vi "exec.vi"(8 "error in (no error)":errorcluster, 10 "context":refnum<class "Context.lvclass">, 11 "Start in":refnum<class "Start.lvclass">) -> (0 "error out":errorcluster, 2 "context 2":refnum<class "Context.lvclass">, 3 "Start out":refnum<class "Start.lvclass">)   [LabVIEW 2013, in "Start.lvclass"]
uses:
  Start.lvclass
  Context/Context.lvclass
  Start.lvclass/Start.ctl
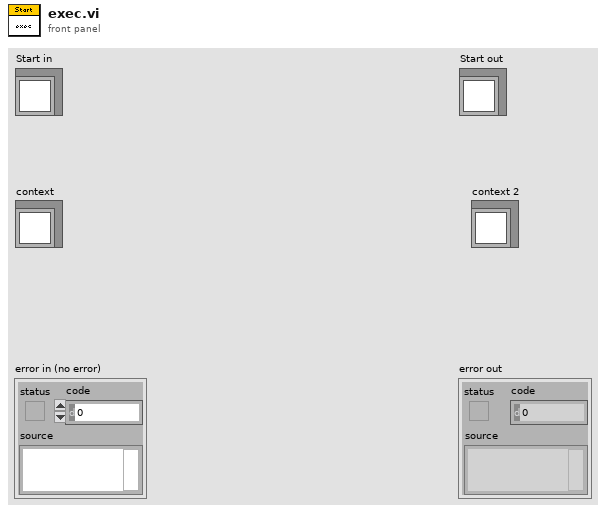
[diagram p1: front panel]
types:
  T1 = typedef "ILCAppConfig.ctl" = cluster{"ILCConfig":T2, "SerialConfig":T5, "Application Timing":T7}
  T2 = typedef "ILCCommon.lvlib/ILCConfiguration.lvlib/ILCConfig.ctl" = cluster{"Input Channels":T3, "Scan Rate (Hz) ":T4, "ADC PGA Gain":u8}
  T3 = typedef "ILCCommon.lvlib/ILCConfiguration.lvlib/InputChannels.ctl" = enum16{"Channel 0", "3 Channels", "5 Channels"}
  T4 = typedef "ILCCommon.lvlib/ILCConfiguration.lvlib/ScanRate_Hz_MultichannelOptions.ctl" = enum16{"50", "60", "100", "120", "200", "240", "300", "400", "480", "600", "1200", "2400", "4800"}
  T5 = typedef "SerialProtocols.lvlib/SerialConfig.ctl" = cluster{"VISA resource name":refnum<visa-resource-name>, "Baud Rate":u32, "Data Bits":u16, "Parity":enum16{"None", "Odd", "Even", "Mark", "Space"}, "Stop Bits":u16, "Flow Control":u16, "Timeout (ms)":u32, "Serial Protocol":T6}
  T6 = typedef "SerialProtocols.lvlib/SerialProtocol.ctl" = enum16{"RS232", "RS485", "SerialSimulator"}
  T7 = typedef "Application.lvlib/ApplicationTiming.ctl" = cluster{"Loop Period (ms)":u16}
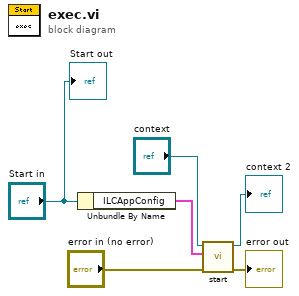
[diagram p0: block diagram]
diagram:
  n1 = Unbundle By Name("Start in") -> ("ILCAppConfig"=w1:T1)
  n2 = call "start.vi"("error in (no error)"="error in (no error)", "ILCAppConfig"=w1, "Context in"="context") -> ("error out"=→"error out":errorcluster, "Context out"=→"context 2":refnum<class "Context.lvclass">)  [unwired: 7 in]
  "Start out" <- "Start in"
